vi "Register.vi"(8 "error in (no error)":errorcluster, 11 "Test Executive Builder in":refnum<class "Test Executive Builder.lvclass">) -> (0 "error out":errorcluster, 3 "Test Executive Builder out":refnum<class "Test Executive Builder.lvclass">)   [LabVIEW 2019, in "Test Executive Builder.lvclass"]
uses:
  <vilib>/gpm_packages/@cs/Test-executive-builder/Example/Application/Test Executive Builder/Test Executive Builder/Test Executive Builder.lvclass
  C:/Program Files/National Instruments/LabVIEW 2019/vi.lib/gpm_packages/@cs/mva-core/Source/IObserver/IObserver/IObserver.lvclass
  <vilib>/gpm_packages/@cs/Test-executive-builder/Source/Test Executive Builder Model/Test Executive Builder Model Messages/Load Test Executive Msg/Load Test Executive Msg.lvclass
  C:/Program Files/National Instruments/LabVIEW 2019/vi.lib/gpm_packages/@cs/transport/Source/Concrete/ActorMessageTransport/Notification Msg/Notification Msg.lvclass
  <vilib>/gpm_packages/@cs/mva-core/Source/SubscriptionPolicy/BasicSubscription/BasicSubscription.lvclass
  C:/Program Files/National Instruments/LabVIEW 2019/vi.lib/gpm_packages/@cs/mva-core/Source/IMediator/ISubscriptionPolicy/ISubscriptionPolicy.lvclass
  <vilib>/gpm_packages/@cs/Test-executive-builder/Source/Test Executive Builder Model/Test Executive Builder Model Messages/Insert While Loop Msg/Insert While Loop Msg.lvclass
  <vilib>/gpm_packages/@cs/Test-executive-builder/Source/Application Dependencies/Insert While Loop.ctl
  <vilib>/gpm_packages/@cs/Test-executive-builder/Source/Test Executive Builder Model/Test Executive Builder Model Messages/Insert For Loop Msg/Insert For Loop Msg.lvclass
  <vilib>/gpm_packages/@cs/Test-executive-builder/Source/Application Dependencies/Insert For Loop.ctl
  <vilib>/gpm_packages/@cs/Test-executive-builder/Source/Test Executive Builder Model/Test Executive Builder Model Messages/Insert Stop Loop Msg/Insert Stop Loop Msg.lvclass
  <vilib>/gpm_packages/@cs/Test-executive-builder/Source/Application Dependencies/Insert Stop Loop.ctl
  <vilib>/gpm_packages/@cs/Test-executive-builder/Source/Test Executive Builder Model/Test Executive Builder Model Messages/Insert Test Step Msg/Insert Test Step Msg.lvclass
  <vilib>/gpm_packages/@cs/Test-executive-builder/Source/Application Dependencies/Insert Test Step.ctl
  <vilib>/gpm_packages/@cs/Test-executive-builder/Source/Test Executive Builder Model/Test Executive Builder Model Messages/Insert Subroutine Msg/Insert Subroutine Msg.lvclass
  <vilib>/gpm_packages/@cs/Test-executive-builder/Source/Application Dependencies/Insert Subroutine.ctl
  <vilib>/gpm_packages/@cs/Test-executive-builder/Source/Test Executive Builder Model/Test Executive Builder Model Messages/Insert Subsequence Msg/Insert Subsequence Msg.lvclass
  <vilib>/gpm_packages/@cs/Test-executive-builder/Source/Application Dependencies/Insert Subsequence.ctl
  <vilib>/gpm_packages/@cs/Test-executive-builder/Source/Test Executive Builder Model/Test Executive Builder Model Messages/Insert Conditional Msg/Insert Conditional Msg.lvclass
  <vilib>/gpm_packages/@cs/Test-executive-builder/Source/Application Dependencies/Insert Conditional.ctl
  <vilib>/gpm_packages/@cs/Test-executive-builder/Source/Test Executive Builder Model/Test Executive Builder Model Messages/Remove Element Msg/Remove Element Msg.lvclass
  <vilib>/gpm_packages/@cs/Test-executive-builder/Source/Test Executive Builder Model/Test Executive Builder Model Messages/Move or Copy Element Msg/Move or Copy Element Msg.lvclass
  <vilib>/gpm_packages/@cs/Test-executive-builder/Source/Application Dependencies/Move or Copy Element.ctl
  <vilib>/gpm_packages/@cs/Test-executive-builder/Source/Test Executive Builder Model/Test Executive Builder Model Messages/Save Test Executive Msg/Save Test Executive Msg.lvclass
  <vilib>/gpm_packages/@cs/Test-executive-builder/Source/Test Executive Builder Model/Test Executive Builder Model Messages/Clear Test Executive Msg/Clear Test Executive Msg.lvclass
  <vilib>/gpm_packages/@cs/Test-executive-builder/Source/Test Executive Builder Model/Test Executive Builder Model Messages/Create Test Executive Msg/Create Test Executive Msg.lvclass
  <vilib>/gpm_packages/@cs/Test-executive-builder/Source/Application Dependencies/Create Test Executive.ctl
  <vilib>/gpm_packages/@cs/Test-executive-builder/Source/Test Executive Builder Model/Test Executive Builder Model Messages/Handle Double Click on Element Msg/Handle Double Click on Element Msg.lvclass
  <vilib>/gpm_packages/@cs/Test-executive-builder/Source/Test Executive Builder Model/Test Executive Builder Model Messages/Drop Element Msg/Drop Element Msg.lvclass
  <vilib>/gpm_packages/@cs/Test-executive-builder/Source/Application Dependencies/Drop Element.ctl
  <vilib>/gpm_packages/@cs/Test-executive-builder/Source/Application Dependencies/Insert Case Structure.ctl
  <vilib>/gpm_packages/@cs/Test-executive-builder/Source/Test Executive Builder Model/Test Executive Builder Model Messages/Insert Case Structure Msg/Insert Case Structure Msg.lvclass
  <vilib>/gpm_packages/@cs/Test-executive-builder/Source/Application Dependencies/Insert Halt.ctl
  <vilib>/gpm_packages/@cs/Test-executive-builder/Source/Test Executive Builder Model/Test Executive Builder Model Messages/Insert Halt Msg/Insert Halt Msg.lvclass
  <vilib>/gpm_packages/@cs/Test-executive-builder/Source/Application Dependencies/Create Paramaterized Executive.ctl
  <vilib>/gpm_packages/@cs/Test-executive-builder/Source/Test Executive Builder Model/Test Executive Builder Model Messages/Create Paramaterized Executive Msg/Create Paramaterized Executive Msg.lvclass
  <vilib>/gpm_packages/@cs/Test-executive-builder/Source/Application Dependencies/Save As Test Executive.ctl
  <vilib>/gpm_packages/@cs/Test-executive-builder/Source/Test Executive Builder Model/Test Executive Builder Model Messages/Save As Test Executive Msg/Save As Test Executive Msg.lvclass
  <vilib>/gpm_packages/@cs/Test-executive-builder/Source/Test Executive Builder Model/Test Executive Builder Model Messages/Mass Relink Msg/Mass Relink Msg.lvclass
  <vilib>/gpm_packages/@cs/Test-executive-builder/Source/Test Executive Builder Model/Test Executive Builder Model Messages/Insert Parallel Msg/Insert Parallel Msg.lvclass
  <vilib>/gpm_packages/@cs/Test-executive-builder/Source/Application Dependencies/Insert Parallel.ctl
  <vilib>/gpm_packages/@cs/mva-core/Source/SubscriptionPolicy/BasicSubscription/BasicSubscription.lvclass/BasicSubscription.ctl
  <vilib>/ActorFramework/Actor/Actor.lvclass/Actor.ctl
  <vilib>/ActorFramework/Message Enqueuer/Message Enqueuer.lvclass/Message Enqueuer.ctl
  <vilib>/gpm_packages/@cs/transport/Source/Concrete/ActorMessageTransport/ActorMessageTransport.lvclass/ActorMessageTransport.ctl
  <vilib>/gpm_packages/@cs/mva-core/Source/IMediator/SubscriptionRequest/SubscriptionRequest.lvclass/SubscriptionRequest.ctl
  <vilib>/gpm_packages/@cs/mva-core/Source/IObserver/IObserver Messages/Subscribe Msg/Subscribe Msg.lvclass/Subscribe Msg.ctl
  <vilib>/gpm_packages/@cs/Test-executive-builder/Example/Application/Test Executive Builder/Test Executive Builder/Test Executive Builder.lvclass/Test Executive Builder.ctl
  <vilib>/gpm_packages/@cs/mva-core/Source/IMediator/SubscriptionRequest/Pack Subscription Request.vi
  <vilib>/gpm_packages/@cs/mva-core/Source/IObserver/IObserver Messages/Subscribe Msg/Send Subscribe.vi
  <vilib>/ActorFramework/Actor/Read Self Enqueuer.vi
  <vilib>/gpm_packages/@cs/transport/Source/Concrete/ActorMessageTransport/Construct Actor Message Transport.vi
  <vilib>/ActorFramework/Message Enqueuer/Enqueue.vi
  <vilib>/ActorFramework/Message Enqueuer/Init from Existing Queue.vi
  <vilib>/ActorFramework/Message Enqueuer/Equals Not A Refnum.vi
  <vilib>/gpm_packages/@cs/mva-core/Source/IObserver/IObserver/IObserver.lvclass
  C:/Program Files/National Instruments/LabVIEW 2019/vi.lib/ActorFramework/Actor/Actor.lvclass
  <vilib>/gpm_packages/@cs/transport/Source/Concrete/ActorMessageTransport/ActorMessageTransport.lvclass
  C:/Program Files/National Instruments/LabVIEW 2019/vi.lib/gpm_packages/@cs/transport/Source/ITransport/ITransport.lvclass
  <vilib>/gpm_packages/@cs/mva-core/Source/IObserver/IObserver Messages/Subscribe Msg/Subscribe Msg.lvclass
  C:/Program Files/National Instruments/LabVIEW 2019/vi.lib/ActorFramework/Message/Message.lvclass
  <vilib>/Utility/error.llb/Error Cluster From Error Code.vi
  <vilib>/gpm_packages/@cs/mva-core/Source/IMediator/ISubscriptionPolicy/Open Subscription Policy.vi
  <vilib>/ActorFramework/Message Priority Queue/Priority Enqueue.vi
  <vilib>/ActorFramework/Message Enqueuer/Message Enqueuer.lvclass
  <vilib>/gpm_packages/@cs/mva-core/Source/IMediator/SubscriptionRequest/SubscriptionRequest.lvclass
  <vilib>/gpm_packages/@cs/transport/Source/Concrete/ActorMessageTransport/Notification Msg/Notification Msg.lvclass
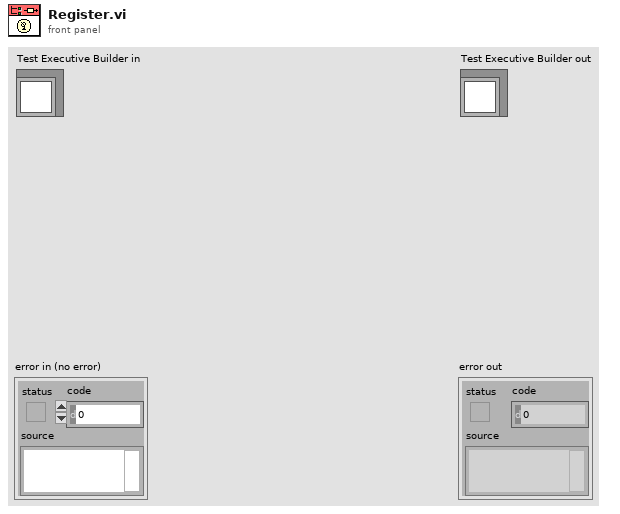
[diagram p1: front panel]
types:
  T1 = typedef "Insert Parallel.ctl" = cluster{"Parent ID":string, "Insertion Index":i32}
  T2 = typedef "Save As Test Executive.ctl" = cluster{"Start Path":path, "Pattern (all files)":string, "Pattern Label":string, "Button Label":string, "Default Name":string, "Prompt":string, "Source File":path, "Delete Source File?":bool}
  T3 = typedef "Create Paramaterized Executive.ctl" = cluster{"Source Folder Path":path, "Source File Name with Extension":string, "Attribute Name Blacklist":string[], "Sink Folder Path":path, "Sink File Name with Extension":string}
  T4 = typedef "Insert Halt.ctl" = cluster{"Parent ID":string, "Insertion Index":i32}
  T5 = typedef "Insert Case Structure.ctl" = cluster{"Parent ID":string, "Insertion Index":i32}
  T6 = typedef "Drop Element.ctl" = cluster{"Parent ID":string, "Insertion Index":i32, "Tag":string, "Ctrl":bool}
  T7 = typedef "Create Test Executive.ctl" = cluster{"Folder Path":path, "File Name with Extension":string}
  T8 = typedef "Move or Copy Element.ctl" = cluster{"Parent ID":string, "Insertion Index":i32, "Tag":string, "Ctrl":bool}
  T9 = typedef "Insert Conditional.ctl" = cluster{"Parent ID":string, "Insertion Index":i32}
  T10 = typedef "Insert Subsequence.ctl" = cluster{"Parent ID":string, "Insertion Index":i32}
  T11 = typedef "Insert Subroutine.ctl" = cluster{"Parent ID":string, "Insertion Index":i32, "Path":path}
  T12 = typedef "Insert Test Step.ctl" = cluster{"Parent ID":string, "Insertion Index":i32, "Test Step":string}
  T13 = typedef "Insert Stop Loop.ctl" = cluster{"Parent ID":string, "Insertion Index":i32}
  T14 = typedef "Insert For Loop.ctl" = cluster{"Parent ID":string, "Insertion Index":i32, "Iterations":i32}
  T15 = typedef "Insert While Loop.ctl" = cluster{"Parent ID":string, "Insertion Index":i32}
  T16 = typedef "IMediator.lvlib/ISubscriptionPolicy.lvclass/ISubscriptionPolicy Reference.ctl" = refnum<data-value>
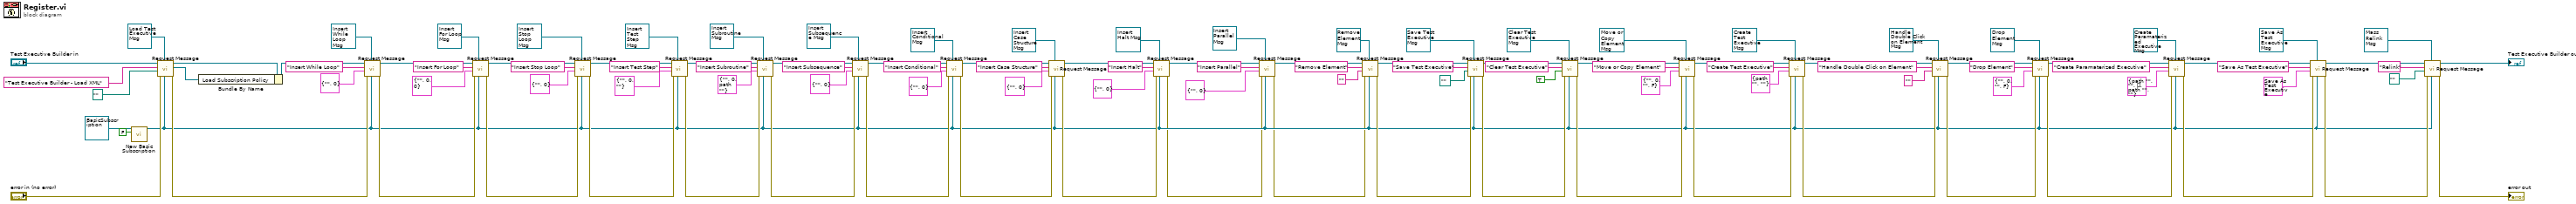
[diagram p0: block diagram]
diagram:
  n1 = call <vilib>:"New Basic Subscription.vi"("Ignore Past Updates? (F)"=FALSE, "BasicSubscription In"=refnum<class "BasicSubscription.lvclass"> refnum ("SubscriptionPolicy.lvlib:BasicSubscription.lvclass")) -> ("BasicSubscription Out"=w3:refnum<class "BasicSubscription.lvclass">)  [unwired: 9 in]
  n2 = call <vilib>:"Request Message.vi"("Configured SubscriptionPolicy"=w3, "Desired Notification Msg"=refnum<class "Load Test Executive Msg.lvclass"> refnum ("Test Executive Builder Model.lvlib:Load Test Executive Msg.lvclass"), "error in (no error)"="error in (no error)", "Data Type"=path "", "Datum Name"="Test Executive Builder - Load XML", "IObserver in"="Test Executive Builder in") -> ("error out"=w101:errorcluster, "Subscription Policy"=w104:T16, "IObserver out"=w105:refnum<class "Test Executive Builder.lvclass">)  [unwired: 3 in]
  n3 = Bundle By Name(cluster=w105, "Load Subscription Policy"=w104) -> (w103:refnum<class "Test Executive Builder.lvclass">)
  n4 = call <vilib>:"Request Message.vi"("Configured SubscriptionPolicy"=w3, "Desired Notification Msg"=refnum<class "Insert While Loop Msg.lvclass"> refnum ("Test Executive Builder Model.lvlib:Insert While Loop Msg.lvclass"), "error in (no error)"=w101, "Data Type"=T15 {"Parent ID"="", "Insertion Index"=0} ("Insert While Loop"), "Datum Name"="Insert While Loop", "IObserver in"=w103) -> ("error out"=w94:errorcluster, "IObserver out"=w95:refnum<class "Test Executive Builder.lvclass">)  [unwired: 3 in, 1 out]
  n5 = call <vilib>:"Request Message.vi"("Configured SubscriptionPolicy"=w3, "Desired Notification Msg"=refnum<class "Insert For Loop Msg.lvclass"> refnum ("Test Executive Builder Model.lvlib:Insert For Loop Msg.lvclass"), "error in (no error)"=w94, "Data Type"=T14 {"Parent ID"="", "Insertion Index"=0, "Iterations"=0} ("Insert For Loop"), "Datum Name"="Insert For Loop", "IObserver in"=w95) -> ("error out"=w89:errorcluster, "IObserver out"=w90:refnum<class "Test Executive Builder.lvclass">)  [unwired: 3 in, 1 out]
  n6 = call <vilib>:"Request Message.vi"("Configured SubscriptionPolicy"=w3, "Desired Notification Msg"=refnum<class "Insert Stop Loop Msg.lvclass"> refnum ("Test Executive Builder Model.lvlib:Insert Stop Loop Msg.lvclass"), "error in (no error)"=w89, "Data Type"=T13 {"Parent ID"="", "Insertion Index"=0} ("Insert Stop Loop"), "Datum Name"="Insert Stop Loop", "IObserver in"=w90) -> ("error out"=w84:errorcluster, "IObserver out"=w85:refnum<class "Test Executive Builder.lvclass">)  [unwired: 3 in, 1 out]
  n7 = call <vilib>:"Request Message.vi"("Configured SubscriptionPolicy"=w3, "Desired Notification Msg"=refnum<class "Insert Test Step Msg.lvclass"> refnum ("Test Executive Builder Model.lvlib:Insert Test Step Msg.lvclass"), "error in (no error)"=w84, "Data Type"=T12 {"Parent ID"="", "Insertion Index"=0, "Test Step"=""} ("Insert Test Step"), "Datum Name"="Insert Test Step", "IObserver in"=w85) -> ("error out"=w79:errorcluster, "IObserver out"=w80:refnum<class "Test Executive Builder.lvclass">)  [unwired: 3 in, 1 out]
  n8 = call <vilib>:"Request Message.vi"("Configured SubscriptionPolicy"=w3, "Desired Notification Msg"=refnum<class "Insert Subroutine Msg.lvclass"> refnum ("Test Executive Builder Model.lvlib:Insert Subroutine Msg.lvclass"), "error in (no error)"=w79, "Data Type"=T11 {"Parent ID"="", "Insertion Index"=0, "Path"=path ""} ("Insert Subroutine"), "Datum Name"="Insert Subroutine", "IObserver in"=w80) -> ("error out"=w74:errorcluster, "IObserver out"=w75:refnum<class "Test Executive Builder.lvclass">)  [unwired: 3 in, 1 out]
  n9 = call <vilib>:"Request Message.vi"("Configured SubscriptionPolicy"=w3, "Desired Notification Msg"=refnum<class "Insert Subsequence Msg.lvclass"> refnum ("Test Executive Builder Model.lvlib:Insert Subsequence Msg.lvclass"), "error in (no error)"=w74, "Data Type"=T10 {"Parent ID"="", "Insertion Index"=0} ("Insert Subsequence"), "Datum Name"="Insert Subsequence", "IObserver in"=w75) -> ("error out"=w69:errorcluster, "IObserver out"=w70:refnum<class "Test Executive Builder.lvclass">)  [unwired: 3 in, 1 out]
  n10 = call <vilib>:"Request Message.vi"("Configured SubscriptionPolicy"=w3, "Desired Notification Msg"=refnum<class "Insert Conditional Msg.lvclass"> refnum ("Test Executive Builder Model.lvlib:Insert Conditional Msg.lvclass"), "error in (no error)"=w69, "Data Type"=T9 {"Parent ID"="", "Insertion Index"=0} ("Insert Conditional"), "Datum Name"="Insert Conditional", "IObserver in"=w70) -> ("error out"=w31:errorcluster, "IObserver out"=w33:refnum<class "Test Executive Builder.lvclass">)  [unwired: 3 in, 1 out]
  n11 = call <vilib>:"Request Message.vi"("Configured SubscriptionPolicy"=w3, "Desired Notification Msg"=refnum<class "Insert Case Structure Msg.lvclass"> refnum ("Insert Case Structure Msg.lvclass"), "error in (no error)"=w31, "Data Type"=T5 {"Parent ID"="", "Insertion Index"=0} ("Insert Case Structure"), "Datum Name"="Insert Case Structure", "IObserver in"=w33) -> ("error out"=w26:errorcluster, "IObserver out"=w27:refnum<class "Test Executive Builder.lvclass">)  [unwired: 3 in, 1 out]
  n12 = call <vilib>:"Request Message.vi"("Configured SubscriptionPolicy"=w3, "Desired Notification Msg"=refnum<class "Insert Halt Msg.lvclass"> refnum ("Insert Halt Msg.lvclass"), "error in (no error)"=w26, "Data Type"=T4 {"Parent ID"="", "Insertion Index"=0} ("Insert Halt"), "Datum Name"="Insert Halt", "IObserver in"=w27) -> ("error out"=w2:errorcluster, "IObserver out"=w5:refnum<class "Test Executive Builder.lvclass">)  [unwired: 3 in, 1 out]
  n13 = call <vilib>:"Request Message.vi"("Configured SubscriptionPolicy"=w3, "Desired Notification Msg"=refnum<class "Insert Parallel Msg.lvclass"> refnum ("Insert Parallel Msg.lvclass"), "error in (no error)"=w2, "Data Type"=T1 {"Parent ID"="", "Insertion Index"=0} ("Insert Parallel"), "Datum Name"="Insert Parallel", "IObserver in"=w5) -> ("error out"=w1:errorcluster, "IObserver out"=w4:refnum<class "Test Executive Builder.lvclass">)  [unwired: 3 in, 1 out]
  n14 = call <vilib>:"Request Message.vi"("Configured SubscriptionPolicy"=w3, "Desired Notification Msg"=refnum<class "Remove Element Msg.lvclass"> refnum ("Test Executive Builder Model.lvlib:Remove Element Msg.lvclass"), "error in (no error)"=w1, "Data Type"="", "Datum Name"="Remove Element", "IObserver in"=w4) -> ("error out"=w53:errorcluster, "IObserver out"=w54:refnum<class "Test Executive Builder.lvclass">)  [unwired: 3 in, 1 out]
  n15 = call <vilib>:"Request Message.vi"("Configured SubscriptionPolicy"=w3, "Desired Notification Msg"=refnum<class "Save Test Executive Msg.lvclass"> refnum ("Test Executive Builder Model.lvlib:Save Test Executive Msg.lvclass"), "error in (no error)"=w53, "Data Type"=path "", "Datum Name"="Save Test Executive", "IObserver in"=w54) -> ("error out"=w52:errorcluster, "IObserver out"=w62:refnum<class "Test Executive Builder.lvclass">)  [unwired: 3 in, 1 out]
  n16 = call <vilib>:"Request Message.vi"("Configured SubscriptionPolicy"=w3, "Desired Notification Msg"=refnum<class "Clear Test Executive Msg.lvclass"> refnum ("Test Executive Builder Model.lvlib:Clear Test Executive Msg.lvclass"), "error in (no error)"=w52, "Data Type"=TRUE, "Datum Name"="Clear Test Executive", "IObserver in"=w62) -> ("error out"=w51:errorcluster, "IObserver out"=w61:refnum<class "Test Executive Builder.lvclass">)  [unwired: 3 in, 1 out]
  n17 = call <vilib>:"Request Message.vi"("Configured SubscriptionPolicy"=w3, "Desired Notification Msg"=refnum<class "Move or Copy Element Msg.lvclass"> refnum ("Test Executive Builder Model.lvlib:Move or Copy Element Msg.lvclass"), "error in (no error)"=w51, "Data Type"=T8 {"Parent ID"="", "Insertion Index"=0, "Tag"="", "Ctrl"=FALSE} ("Move or Copy Element"), "Datum Name"="Move or Copy Element", "IObserver in"=w61) -> ("error out"=w48:errorcluster, "IObserver out"=w49:refnum<class "Test Executive Builder.lvclass">)  [unwired: 3 in, 1 out]
  n18 = call <vilib>:"Request Message.vi"("Configured SubscriptionPolicy"=w3, "Desired Notification Msg"=refnum<class "Create Test Executive Msg.lvclass"> refnum ("Test Executive Builder Model.lvlib:Create Test Executive Msg.lvclass"), "error in (no error)"=w48, "Data Type"=T7 {"Folder Path"=path "", "File Name with Extension"=""} ("Create Test Executive"), "Datum Name"="Create Test Executive", "IObserver in"=w49) -> ("error out"=w41:errorcluster, "IObserver out"=w42:refnum<class "Test Executive Builder.lvclass">)  [unwired: 3 in, 1 out]
  n19 = call <vilib>:"Request Message.vi"("Configured SubscriptionPolicy"=w3, "Desired Notification Msg"=refnum<class "Handle Double Click on Element Msg.lvclass"> refnum ("Test Executive Builder Model.lvlib:Handle Double Click on Element Msg.lvclass"), "error in (no error)"=w41, "Data Type"="", "Datum Name"="Handle Double Click on Element", "IObserver in"=w42) -> ("error out"=w36:errorcluster, "IObserver out"=w37:refnum<class "Test Executive Builder.lvclass">)  [unwired: 3 in, 1 out]
  n20 = call <vilib>:"Request Message.vi"("Configured SubscriptionPolicy"=w3, "Desired Notification Msg"=refnum<class "Drop Element Msg.lvclass"> refnum ("Test Executive Builder Model.lvlib:Drop Element Msg.lvclass"), "error in (no error)"=w36, "Data Type"=T6 {"Parent ID"="", "Insertion Index"=0, "Tag"="", "Ctrl"=FALSE} ("Drop Element"), "Datum Name"="Drop Element", "IObserver in"=w37) -> ("error out"=w23:errorcluster, "IObserver out"=w24:refnum<class "Test Executive Builder.lvclass">)  [unwired: 3 in, 1 out]
  n21 = call <vilib>:"Request Message.vi"("Configured SubscriptionPolicy"=w3, "Desired Notification Msg"=refnum<class "Create Paramaterized Executive Msg.lvclass"> refnum ("Create Paramaterized Executive Msg.lvclass"), "error in (no error)"=w23, "Data Type"=T3 {"Source Folder Path"=path "", "Source File Name with Extension"="", "Attribute Name Blacklist"=[], "Sink Folder Path"=path "", "Sink File Name with Extension"=""} ("Create Paramaterized Executive"), "Datum Name"="Create Paramaterized Executive", "IObserver in"=w24) -> ("error out"=w18:errorcluster, "IObserver out"=w19:refnum<class "Test Executive Builder.lvclass">)  [unwired: 3 in, 1 out]
  n22 = call <vilib>:"Request Message.vi"("Configured SubscriptionPolicy"=w3, "Desired Notification Msg"=refnum<class "Save As Test Executive Msg.lvclass"> refnum ("Save As Test Executive Msg.lvclass"), "error in (no error)"=w18, "Data Type"=T2 {"Start Path"=path "", "Pattern (all files)"="", "Pattern Label"="", "Button Label"="", "Default Name"="", "Prompt"="", "Source File"=path "", "Delete Source File?"=FALSE} ("Save As Test Executive"), "Datum Name"="Save As Test Executive", "IObserver in"=w19) -> ("error out"=w10:errorcluster, "IObserver out"=w12:refnum<class "Test Executive Builder.lvclass">)  [unwired: 3 in, 1 out]
  n23 = call <vilib>:"Request Message.vi"("Configured SubscriptionPolicy"=w3, "Desired Notification Msg"=refnum<class "Mass Relink Msg.lvclass"> refnum ("Mass Relink Msg.lvclass"), "error in (no error)"=w10, "Data Type"=path "", "Datum Name"="Relink", "IObserver in"=w12) -> ("error out"=→"error out":errorcluster, "IObserver out"=→"Test Executive Builder out":refnum<class "Test Executive Builder.lvclass">)  [unwired: 3 in, 1 out]
